vi "_PC_MS_SubVI displaySpectrumSignal.vi"(7 "graphRefnum in":T1, 8 "error in (no error)":errorcluster, 11 "newSigInfo":T2) -> (0 "error out":errorcluster, 2 "ydata":sgl[][](array[numeric]))   [LabVIEW 2018]
uses:
  <vilib>/Analysis/baseanly.llb/Mean (DBL).vi
  <vilib>/Analysis/NI_AALBase.lvlib
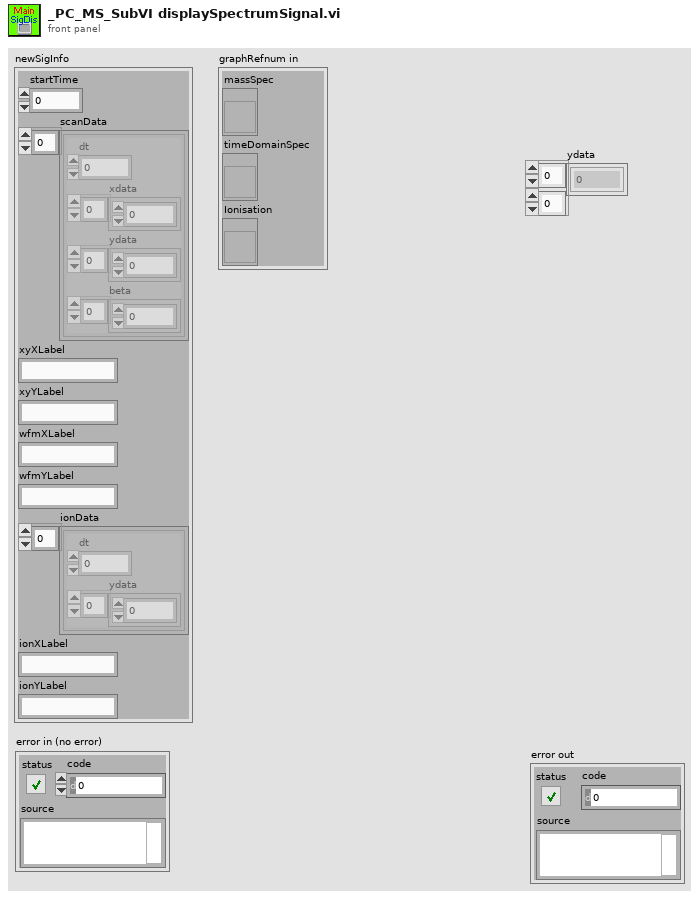
[diagram p1: front panel]
types:
  T1 = cluster{"massSpec":refnum<vi>, "timeDomainSpec":refnum<vi>, "Ionisation":refnum<vi>}
  T2 = cluster{"startTime":dbl, "scanData":cluster{"dt":dbl, "xdata":dbl[], "ydata":sgl[], "beta":dbl[]}[], "xyXLabel":string, "xyYLabel":string, "wfmXLabel":string, "wfmYLabel":string, "ionData":cluster{"dt":dbl, "ydata":sgl[]}[], "ionXLabel":string, "ionYLabel":string}
  T3 = cluster{"dt":dbl, "xdata":dbl[], "ydata":sgl[], "beta":dbl[]}[]
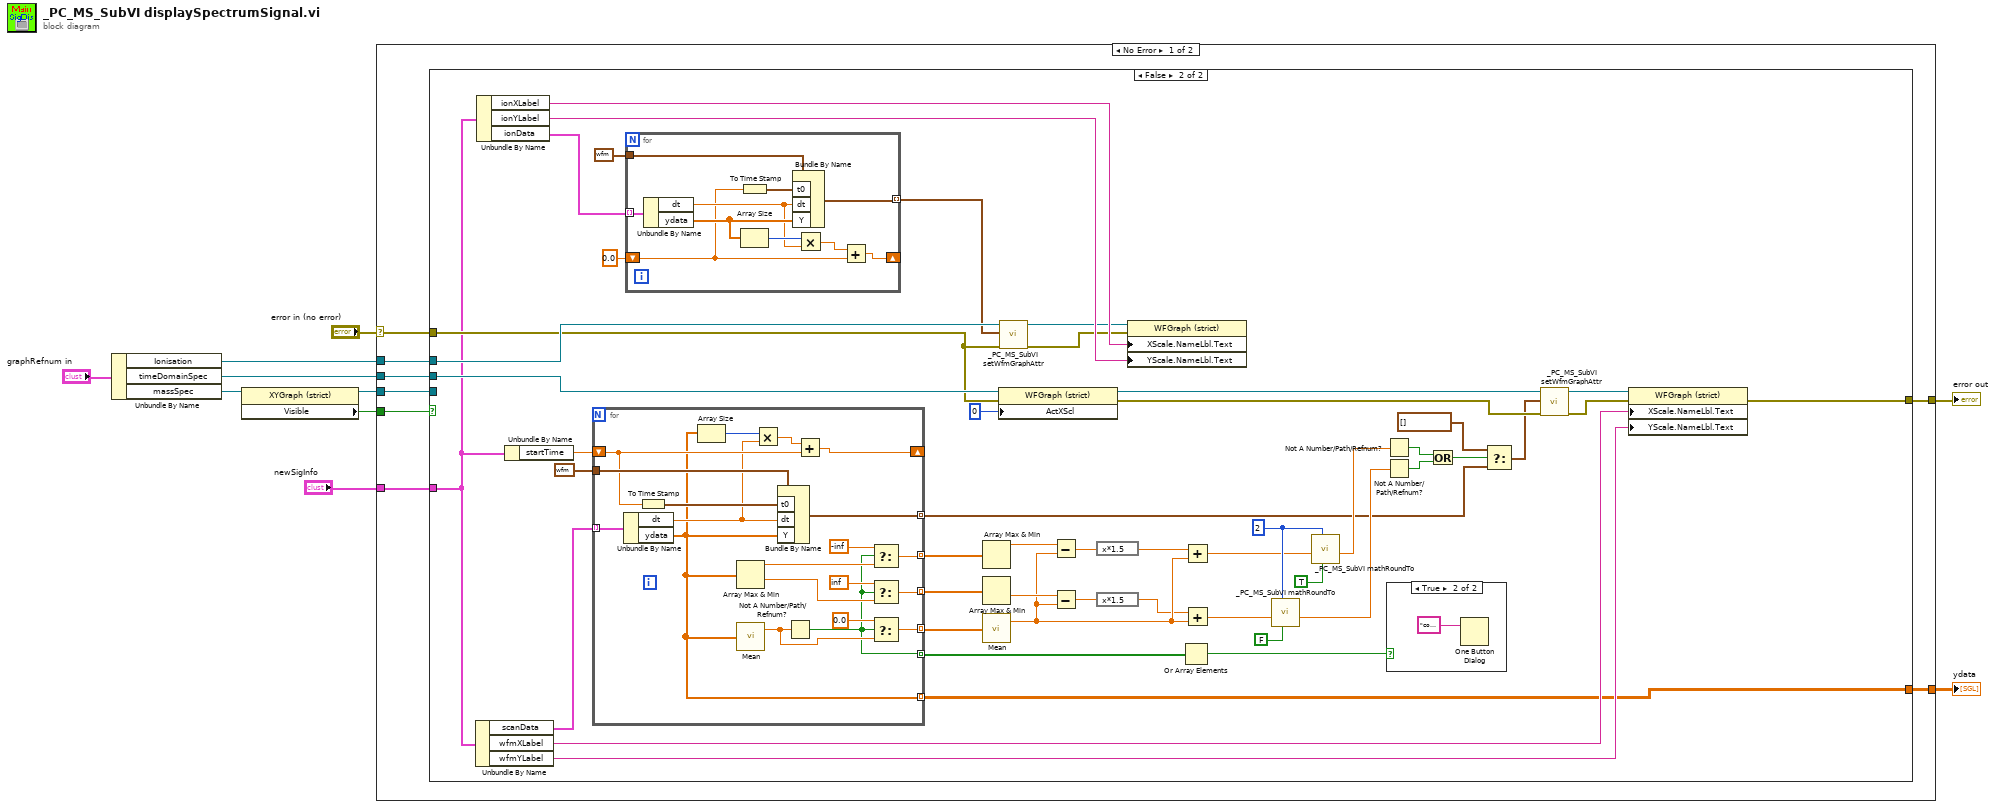
[diagram p0: block diagram]
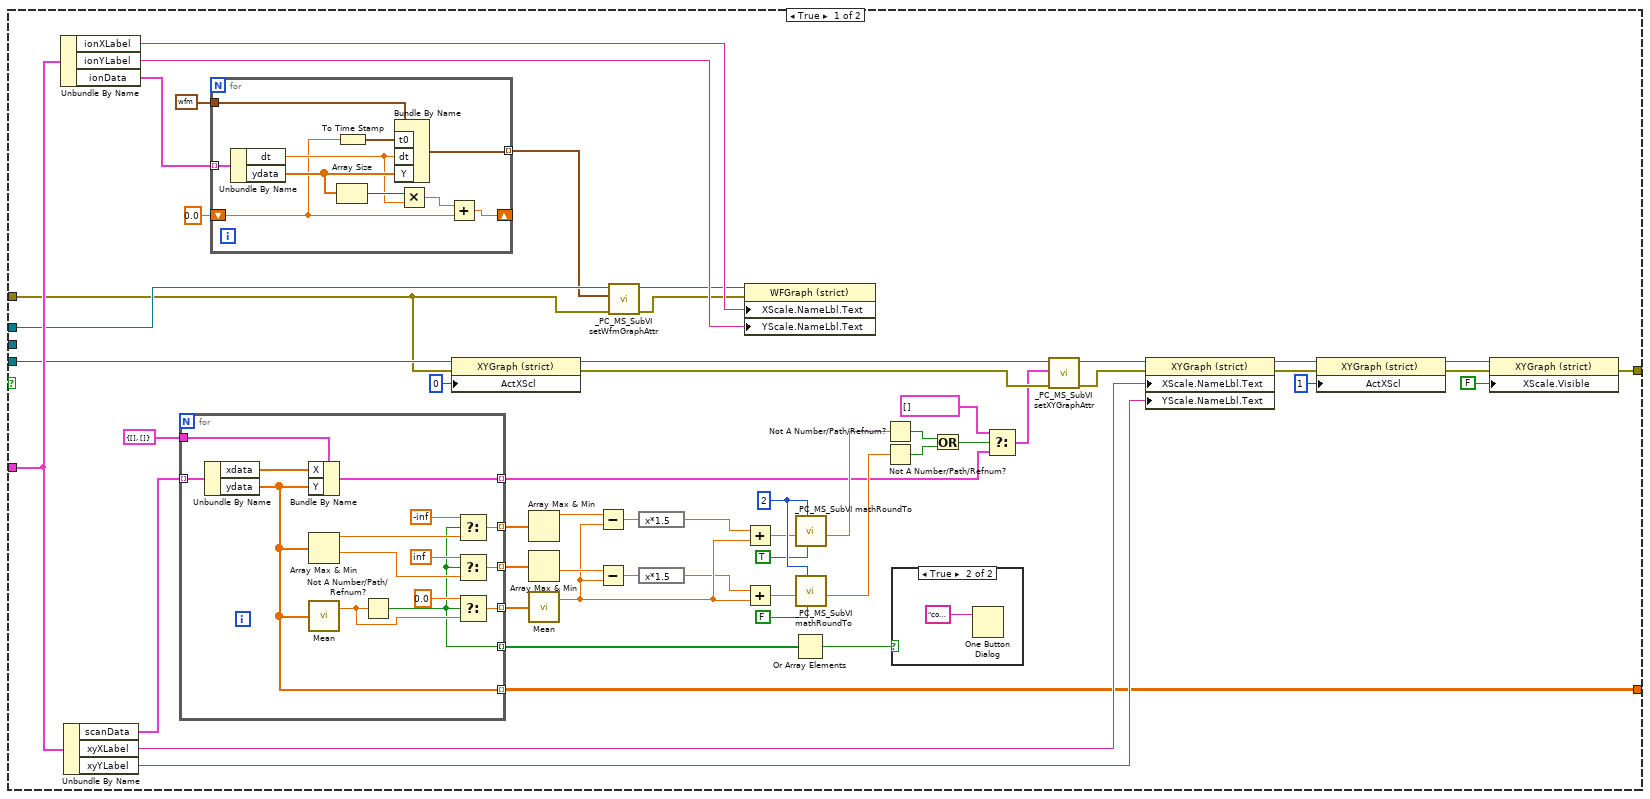
[diagram p2: hidden frame]
diagram:
  n1 = Unbundle By Name("graphRefnum in") -> ("Ionisation"=w3:refnum<vi>, "timeDomainSpec"=w6:refnum<vi>, "massSpec"=w9:refnum<vi>)
  n2 = property class="XYGraph (strict)"(reference=w9) -> (reference out=w7:refnum<vi>, "Visible"=w8:bool)  [unwired: 1 in, 1 out]
  n3 = case shown="No Error" "error in (no error)" {
    selector: "error in (no error)" -> [w14 w179]
    tunnel: w8 -> [w17 _]
    tunnel: w7 -> [w18 _]
    tunnel: w6 -> [w16 _]
    tunnel: [w15 w179] -> w5
    tunnel: w3 -> [w13 _]
    tunnel: "newSigInfo" -> [w12 _]
    tunnel: [w11 _] -> w1
    frame No Error {
      n4 = case shown="False" w17 {
        tunnel: w18 -> [w41 _]
        tunnel: [w50 w115] -> w15
        tunnel: w16 -> [_ w119]
        tunnel: w14 -> [w27 w104]
        tunnel: w13 -> [w29 w108]
        tunnel: w12 -> [w47 w100]
        tunnel: [w38 w110] -> w11
        frame True {
          w71 = 2 ("Digit")
          n5 = Unbundle By Name(w47) -> ("ionXLabel"=w46:string, "ionYLabel"=w45:string, "ionData"=w35:cluster{"dt":dbl, "ydata":sgl[]}[])
          n6 = Unbundle By Name(w47) -> ("scanData"=w44:T3, "xyXLabel"=w40:string, "xyYLabel"=w39:string)
          n7 = for {
            tunnel: [w88] -> w58 mode=indexing
            tunnel: [w85] -> w59 mode=indexing
            tunnel: [w91] -> w57 mode=indexing
            tunnel: w44 -> [w95] mode=indexing
            tunnel: cluster{"X":dbl[], "Y":sgl[]} {"X"=[], "Y"=[]} ("Spectrum in") -> [w98]
            tunnel: [w96] -> w42 mode=indexing
            tunnel: [w94] -> w38 mode=indexing
            tunnel: [w84] -> w20 mode=indexing
            n8 = Unbundle By Name(w95) -> ("xdata"=w97:dbl[], "ydata"=w94:sgl[])
            n9 = Bundle By Name(cluster=w98, "X"=w97, "Y"=w94) -> (w96:cluster{"X":dbl[], "Y":sgl[]})
            n10 = Array Max & Min(array=w94) -> (max value=w86:sgl, min value=w90:sgl)  [unwired: 2 out]
            n11 = call-poly <vilib>:"Mean.vi"("X"=w94) -> ("mean"=w92:dbl)  [unwired: 1 out]
            n12 = Not A Number/Path/Refnum?(number/path/refnum=w92) -> (NaN/Path/Refnum?=w84:bool)
            n13 = Select(t=sgl -inf, s=w84, f=w86) -> (s? t:f=w85:sgl)
            n14 = Select(t=sgl inf, s=w84, f=w90) -> (s? t:f=w88:sgl)
            n15 = Select(t=0.0, s=w84, f=w92) -> (s? t:f=w91:dbl)
          }
          n16 = for {
            tunnel: w35 -> [w81] mode=indexing
            tunnel: waveform(sgl) {"t0"=timestamp(0 s since 1904-01-01), "dt"=1.0, "Y"=[]} -> [w83]
            tunnel: [w80] -> w28 mode=indexing
            shift-right: [w74] -> _
            shift-left: 0.0 ("startTime") -> [w75]
            n17 = Unbundle By Name(w81) -> ("dt"=w76:dbl, "ydata"=w77:sgl[])
            n18 = Array Size(array=w77) -> (size(s)=w79:i32)
            n19 = To Time Stamp(1:w75) -> (0:w82:timestamp)
            n20 = Bundle By Name(cluster=w83, "t0"=w82, "dt"=w76, "Y"=w77) -> (w80:waveform(sgl))
            n21 = Multiply(x=w79, y=w76) -> (x*y=w78:dbl)
            n22 = Add(x=w78, y=w75) -> (x+y=w74:dbl)
          }
          n23 = property class="XYGraph (strict)"(reference=w41, error in=w27, "ActXScl"=0 ("Active X Scale")) -> (reference out=w34:refnum<vi>, error out=w32:errorcluster)
          n24 = Array Max & Min(array=w59) -> (max value=w70:sgl)  [unwired: 3 out]
          n25 = Array Max & Min(array=w58) -> (min value=w69:sgl)  [unwired: 3 out]
          n26 = call-poly <vilib>:"Mean.vi"("X"=w57) -> ("mean"=w66:dbl)  [unwired: 1 out]
          n27 = Subtract(x=w70, y=w66) -> (x-y=w68:dbl)
          n28 = Subtract(x=w69, y=w66) -> (x-y=w67:dbl)
          n29 = call "_PC_MS_SubVI setWfmGraphAttr.vi"("error in (no error)"=w27, "plotValue"=w28, "graph in"=w29) -> ("error out"=w25:errorcluster, "graph out"=w26:refnum<vi>)  [unwired: 7 in]
          n30 = expression code="x*1.5"(w68) -> (w64:dbl)
          n31 = expression code="x*1.5"(w67) -> (w65:dbl)
          n32 = property class="WFGraph (strict)"(reference=w26, error in=w25, "XScale.NameLbl.Text"=w46, "YScale.NameLbl.Text"=w45) -> ()  [unwired: 2 out]
          n33 = Add(x=w64, y=w66) -> (x+y=w63:dbl)
          n34 = Add(x=w65, y=w66) -> (x+y=w62:dbl)
          n35 = Or Array Elements(Boolean array=w20) -> (logical OR=w19:bool)
          n36 = call "_PC_MS_SubVI mathRoundTo.vi"("Up/Down"=TRUE, "Digit"=w71, "Numeric"=w63) -> ("Round to"=w54:dbl)  [unwired: 8 in]
          n37 = call "_PC_MS_SubVI mathRoundTo.vi"("Up/Down"=FALSE, "Digit"=w71, "Numeric"=w62) -> ("Round to"=w53:dbl)  [unwired: 8 in]
          n38 = Not A Number/Path/Refnum?(number/path/refnum=w54) -> (NaN/Path/Refnum?=w56:bool)
          n39 = Not A Number/Path/Refnum?(number/path/refnum=w53) -> (NaN/Path/Refnum?=w55:bool)
          n40 = case shown="True" w19 {
            frame False {
            }
            frame True {
              n41 = One Button Dialog(message="contains \"Not A Number\"") -> ()  [unwired: 1 in, 1 out]
            }
          }
          n42 = Or(x=w56, y=w55) -> (x .or. y?=w52:bool)
          n43 = Select(t=cluster{"X":dbl[], "Y":sgl[]}[] [], s=w52, f=w42) -> (s? t:f=w30:cluster{"X":dbl[], "Y":sgl[]}[])
          n44 = call "_PC_MS_SubVI setXYGraphAttr.vi"("error in (no error)"=w32, "plot value"=w30, "graph in"=w34) -> ("error out"=w31:errorcluster, "graph out"=w33:refnum<vi>)  [unwired: 7 in]
          n45 = property class="XYGraph (strict)"(reference=w33, error in=w31, "XScale.NameLbl.Text"=w40, "YScale.NameLbl.Text"=w39) -> (reference out=w49:refnum<vi>, error out=w48:errorcluster)
          n46 = property class="XYGraph (strict)"(reference=w49, error in=w48, "ActXScl"=1 ("Active X Scale")) -> (reference out=w23:refnum<vi>, error out=w24:errorcluster)
          n47 = property class="XYGraph (strict)"(reference=w23, error in=w24, "XScale.Visible"=FALSE ("X Scale.Visible")) -> (error out=w50:errorcluster)  [unwired: 1 out]
        }
        frame False {
          w146 = 2 ("Digit")
          n48 = Unbundle By Name(w100) -> ("scanData"=w123:T3, "wfmXLabel"=w122:string, "wfmYLabel"=w121:string)
          n49 = Unbundle By Name(w100) -> ("ionXLabel"=w125:string, "ionYLabel"=w124:string, "ionData"=w101:cluster{"dt":dbl, "ydata":sgl[]}[])
          n50 = Unbundle By Name(w100) -> ("startTime"=w99:dbl)
          n51 = for {
            tunnel: [w160] -> w133 mode=indexing
            tunnel: [w161] -> w134 mode=indexing
            tunnel: [w162] -> w132 mode=indexing
            tunnel: w123 -> [w178] mode=indexing
            tunnel: waveform(sgl) {"t0"=timestamp(0 s since 1904-01-01), "dt"=1.0, "Y"=[]} ("Waveform") -> [w177]
            tunnel: [w175] -> w113 mode=indexing
            tunnel: [w163] -> w110 mode=indexing
            shift-right: [w173] -> _
            shift-left: w99 -> [w174]
            tunnel: [w159] -> w103 mode=indexing
            n52 = Unbundle By Name(w178) -> ("dt"=w171:dbl, "ydata"=w163:sgl[])
            n53 = To Time Stamp(1:w174) -> (0:w176:timestamp)
            n54 = Array Size(array=w163) -> (size(s)=w172:i32)
            n55 = Array Max & Min(array=w163) -> (max value=w164:sgl, min value=w167:sgl)  [unwired: 2 out]
            n56 = call-poly <vilib>:"Mean.vi"("X"=w163) -> ("mean"=w168:dbl)  [unwired: 1 out]
            n57 = Multiply(x=w172, y=w171) -> (x*y=w170:dbl)
            n58 = Bundle By Name(cluster=w177, "t0"=w176, "dt"=w171, "Y"=w163) -> (w175:waveform(sgl))
            n59 = Not A Number/Path/Refnum?(number/path/refnum=w168) -> (NaN/Path/Refnum?=w159:bool)
            n60 = Add(x=w170, y=w174) -> (x+y=w173:dbl)
            n61 = Select(t=sgl -inf, s=w159, f=w164) -> (s? t:f=w161:sgl)
            n62 = Select(t=sgl inf, s=w159, f=w167) -> (s? t:f=w160:sgl)
            n63 = Select(t=0.0, s=w159, f=w168) -> (s? t:f=w162:dbl)
          }
          n64 = for {
            tunnel: w101 -> [w156] mode=indexing
            tunnel: waveform(sgl) {"t0"=timestamp(0 s since 1904-01-01), "dt"=1.0, "Y"=[]} -> [w158]
            tunnel: [w155] -> w105 mode=indexing
            shift-right: [w149] -> _
            shift-left: 0.0 ("startTime") -> [w150]
            n65 = Unbundle By Name(w156) -> ("dt"=w151:dbl, "ydata"=w152:sgl[])
            n66 = Array Size(array=w152) -> (size(s)=w154:i32)
            n67 = To Time Stamp(1:w150) -> (0:w157:timestamp)
            n68 = Bundle By Name(cluster=w158, "t0"=w157, "dt"=w151, "Y"=w152) -> (w155:waveform(sgl))
            n69 = Multiply(x=w154, y=w151) -> (x*y=w153:dbl)
            n70 = Add(x=w153, y=w150) -> (x+y=w149:dbl)
          }
          n71 = Array Max & Min(array=w134) -> (max value=w145:sgl)  [unwired: 3 out]
          n72 = Array Max & Min(array=w133) -> (min value=w144:sgl)  [unwired: 3 out]
          n73 = call-poly <vilib>:"Mean.vi"("X"=w132) -> ("mean"=w141:dbl)  [unwired: 1 out]
          n74 = property class="WFGraph (strict)"(reference=w119, error in=w104, "ActXScl"=0 ("Active X Scale")) -> (reference out=w120:refnum<vi>, error out=w118:errorcluster)
          n75 = call "_PC_MS_SubVI setWfmGraphAttr.vi"("error in (no error)"=w104, "plotValue"=w105, "graph in"=w108) -> ("error out"=w106:errorcluster, "graph out"=w107:refnum<vi>)  [unwired: 7 in]
          n76 = Subtract(x=w145, y=w141) -> (x-y=w143:dbl)
          n77 = Subtract(x=w144, y=w141) -> (x-y=w142:dbl)
          n78 = expression code="x*1.5"(w143) -> (w139:dbl)
          n79 = expression code="x*1.5"(w142) -> (w140:dbl)
          n80 = property class="WFGraph (strict)"(reference=w107, error in=w106, "XScale.NameLbl.Text"=w125, "YScale.NameLbl.Text"=w124) -> ()  [unwired: 2 out]
          n81 = Or Array Elements(Boolean array=w103) -> (logical OR=w102:bool)
          n82 = Add(x=w139, y=w141) -> (x+y=w138:dbl)
          n83 = Add(x=w140, y=w141) -> (x+y=w137:dbl)
          n84 = call "_PC_MS_SubVI mathRoundTo.vi"("Up/Down"=FALSE, "Digit"=w146, "Numeric"=w137) -> ("Round to"=w128:dbl)  [unwired: 8 in]
          n85 = call "_PC_MS_SubVI mathRoundTo.vi"("Up/Down"=TRUE, "Digit"=w146, "Numeric"=w138) -> ("Round to"=w129:dbl)  [unwired: 8 in]
          n86 = Not A Number/Path/Refnum?(number/path/refnum=w129) -> (NaN/Path/Refnum?=w131:bool)
          n87 = Not A Number/Path/Refnum?(number/path/refnum=w128) -> (NaN/Path/Refnum?=w130:bool)
          n88 = case shown="True" w102 {
            frame False {
            }
            frame True {
              n89 = One Button Dialog(message="contains \"Not A Number\"") -> ()  [unwired: 1 in, 1 out]
            }
          }
          n90 = Or(x=w131, y=w130) -> (x .or. y?=w127:bool)
          n91 = Select(t=waveform(sgl)[] [], s=w127, f=w113) -> (s? t:f=w111:waveform(sgl)[])
          n92 = call "_PC_MS_SubVI setWfmGraphAttr.vi"("error in (no error)"=w118, "plotValue"=w111, "graph in"=w120) -> ("error out"=w116:errorcluster, "graph out"=w117:refnum<vi>)  [unwired: 7 in]
          n93 = property class="WFGraph (strict)"(reference=w117, error in=w116, "XScale.NameLbl.Text"=w122, "YScale.NameLbl.Text"=w121) -> (error out=w115:errorcluster)  [unwired: 1 out]
        }
      }
    }
    frame Error {
    }
  }
  "error out" <- w5
  "ydata" <- w1
